vi "SVT Octave Analysis (N Ch).vi"(0 "scaled signals [EU]":waveform(dbl)[](array[waveform])=[{"t0"=timestamp(0 s since 1904-01-01), "dt"=1.0, "Y"=[]}], 1 "restart averaging (F)":bool, 2 "reset filter (F)":bool, 5 "frequency range":T7={"low band"=enum."16 Hz", "high band"=enum."16000 Hz"}, 9 "dB On (T)":bool=TRUE, 11 "error in (no error)":errorcluster, 12 "averaging type":T8(ring), 13 "exp avg settings":T1={" mode"=enum."Fast", "time constant [ms]"=125.0} {"time constant [ms]" format="%.2f"}, 14 "equal confidence level [dB]":dbl=125.0 format="%.2f") -> (3 "filter settled":bool, 4 "octave spectra":T6(array[cluster]) {"band power" format="%.2f"; "nominal frequencies [Hz]" format="%.2f"}, 6 "unit labels":string[](array[string]), 8 "total band powers":dbl[](array[numeric]) format="%.2f", 10 "octave info":T2[](array[typedef]) {"engineering units" items=["custom..."=0, "V"=1, "A"=21, "C"=30, "pC"=31, "s"=32, "-"=29, "Pa"=2, "N"=20, "g"=3, "m/s^2"=4, "m/s"=5, "m"=6, "mm/s"=12, "mm"=13, "micron/s"=14, "micron"=15, "in/s^2"=7, "in/s"=8, "in"=9, "mil/s"=10, "mil"=11, "rad/s^2"=16, "rad/s"=17, "rad"=18, "deg/s^2"=26, "deg/s"=27, "deg"=28, "RPM"=22, "cycle/s^2"=23, "Hz"=24, "cycle"=25, "strain"=19]; "dB reference" format="%.2e"; "weighting filter" items=["Linear", "A-weighting", "B-weighting", "C-weighting", "ITU-R 468-4", "Dolby", "CCITT", "C-message", "Wb", "Wc", "Wd", "We", "Wf", "Wh", "Wj", "Wk", "Wm", "AES17 20 kHz lowpass", "AES17 40 kHz lowpass", "AES17 20 kHz highpass", "AES17 40 kHz highpass"]}, 15 "error out":errorcluster)   [LabVIEW 2017, in "SoundVib_Octave.lvlib"]
doc: "LabVIEW no longer supports this VI. The SVT Octave Analysis VI is available for compatibility with previous versions of the LabVIEW Sound and Vibration Toolkit. This version of the SVT Octave Analysis VI performs an octave analysis on <B>scaled signal [EU]</B> in accordance with the IEC 1260 standard. This standard has been superseded by the new IEC 61260 standard. If you want to ensure compliance with the latter standard, use the SVT Octave Analysis VI, located on the Octave Analysis palette instead. You can use this polymorphic VI to perform octave analysis on a single channel or on N channels. The data type you wire to the <B>scaled signal [EU]</B> input determines the polymorphic instance to use."
uses:
  <vilib>/addons/Sound and Vibration/svt_Octave/SoundVib_Octave.lvlib
  <vilib>/addons/_NISVFA/_Shared subVIs/Controls/svc_Octave Info.ctl
  <vilib>/addons/_NISVFA/_Shared subVIs/Controls/svc_Octave Standard.ctl
  <vilib>/addons/_NISVFA/_Shared subVIs/Controls/svc_Weighting Filter Text Ring.ctl
  <vilib>/addons/_NISVFA/_Shared subVIs/Controls/svc_Engineering Units Text Ring.ctl
  <vilib>/addons/Sound and Vibration/svt_Octave_2014 standard/SoundVib_Octave_2014 standard.lvlib
panel:
  out "# samples to settle":u64
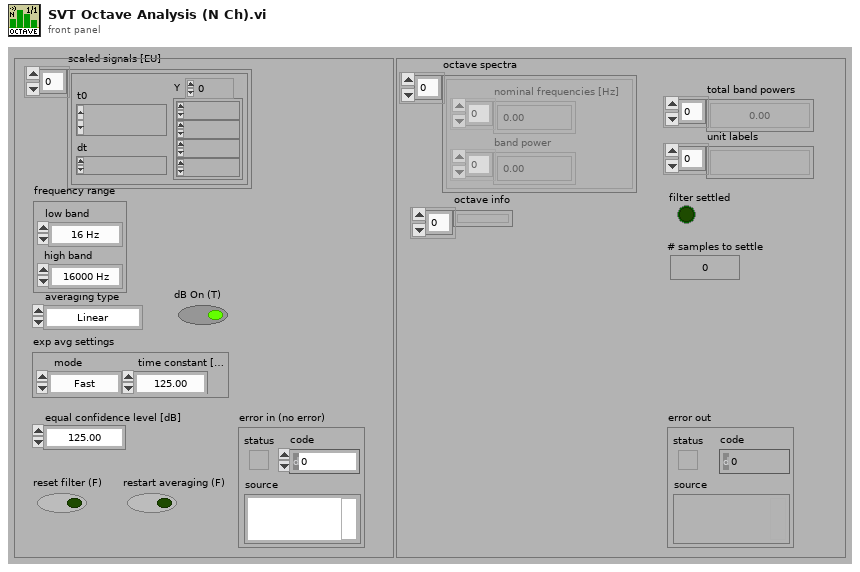
[diagram p1: front panel]
types:
  T1 = cluster{" mode":enum16{"Slow", "Fast", "Impulse", "Custom"}, "time constant [ms]":dbl}
  T2 = typedef "svc_Octave Info.ctl" = cluster{"standard":T3, "bandwidth":enum16{"1 octave", "1/3 octave", "1/6 octave", "1/12 octave", "1/24 octave"}, "low band":i32, "high band":i32, "weighting filter":T4, "dB reference":dbl, "dB On":bool, "unit label":string, "channel name":string, "description":string, "engineering units":T5, "custom label":string, "spectrum type":enum16{"power", "magnitude"}, "spectral density":bool, "filters settled":bool}
  T3 = typedef "svc_Octave Standard.ctl" = enum16{"ANSI S1.11", "IEC 61260"}
  T4 = typedef "svc_Weighting Filter Text Ring.ctl" = u16
  T5 = typedef "svc_Engineering Units Text Ring.ctl" = u16
  T6 = cluster{"nominal frequencies [Hz]":dbl[], "band power":dbl[]}[]
  T7 = cluster{"low band":enum16{"16 Hz", "31.5 Hz", "63 Hz", "125 Hz", "250 Hz", "500 Hz", "1000 Hz", "2000 Hz", "4000 Hz", "8000 Hz", "16000 Hz"}, "high band":enum16{"16 Hz", "31.5 Hz", "63 Hz", "125 Hz", "250 Hz", "500 Hz", "1000 Hz", "2000 Hz", "4000 Hz", "8000 Hz", "16000 Hz"}}
  T8 = enum16{"Linear", "Exponential", "Equal confidence", "Peak"}
  T9 = cluster{"standard":T3, "bandwidth":enum16{"1 octave", "1/3 octave", "1/6 octave", "1/12 octave", "1/24 octave"}}
  T10 = cluster{"dup nominal frequencies [Hz":dbl[], "band power [EU^2 rms]":dbl[]}[]
  T11 = cluster{"nominal frequencies [Hz]":dbl[], "band power [dB EU]":dbl[]}[]
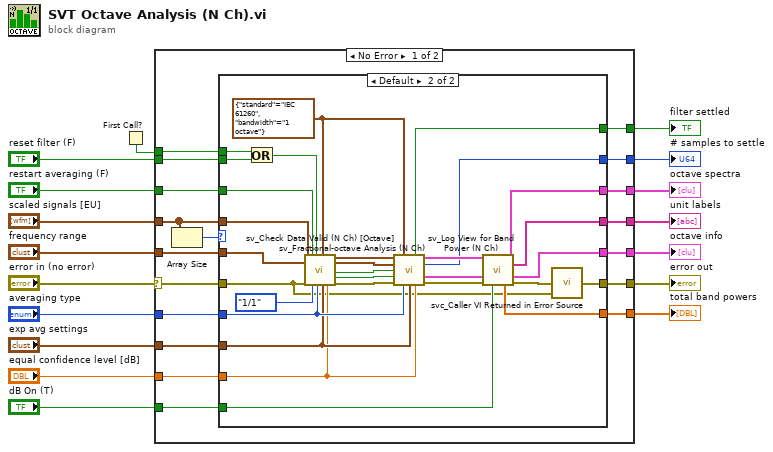
[diagram p0: block diagram]
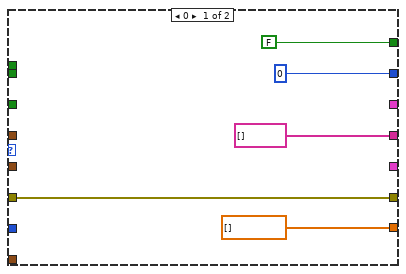
[diagram p2: hidden frame]
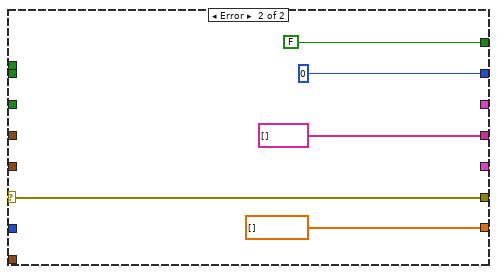
[diagram p3: hidden frame]
diagram:
  n1 = First Call?() -> (First Call?: T/F=w1:bool)
  n2 = case shown="No Error" "error in (no error)" {
    selector: "error in (no error)" -> [w25 w74]
    tunnel: "restart averaging (F)" -> [w35 _]
    tunnel: "frequency range" -> [w34 _]
    tunnel: [w23 FALSE ("settled?")] -> w15
    tunnel: "dB On (T)" -> [w33 _]
    tunnel: "averaging type" -> [w32 _]
    tunnel: "equal confidence level [dB]" -> [w24 _]
    tunnel: "exp avg settings" -> [w31 _]
    tunnel: [w30 dbl[] [] ("total band power(s) [dB EU]")] -> w10
    tunnel: "scaled signals [EU]" -> [w19 _]
    tunnel: [w26 w74] -> w8
    tunnel: [w29 _] -> w7
    tunnel: [w28 string[] [] ("unit labels")] -> w6
    tunnel: [w27 _] -> w5
    tunnel: [w22 u64 0 ("# samples to settle")] -> w3
    tunnel: "reset filter (F)" -> [w21 _]
    tunnel: w1 -> [w20 _]
    frame No Error {
      n3 = Array Size(array=w19) -> (size(s)=w18:i32)
      n4 = case shown="Default" w18 {
        tunnel: w35 -> [_ w69]
        tunnel: w34 -> [_ w68]
        tunnel: w33 -> [_ w63]
        tunnel: w32 -> [_ w61]
        tunnel: w31 -> [_ w60]
        tunnel: [dbl[] [] ("total band power(s) [dB EU]") w59] -> w30
        tunnel: w19 -> [_ w56]
        tunnel: [_ w54] -> w29
        tunnel: [string[] [] ("unit labels") w53] -> w28
        tunnel: [_ w52] -> w27
        tunnel: [w37 w50] -> w26
        tunnel: w25 -> [w37 w41]
        tunnel: w24 -> [_ w48]
        tunnel: [FALSE ("settled?") w45] -> w23
        tunnel: [u64 0 ("# samples to settle") w44] -> w22
        tunnel: w21 -> [_ w43]
        tunnel: w20 -> [_ w42]
        frame 0 {
        }
        frame Default {
          w58 = T9 {"standard"=enum."IEC 61260", "bandwidth"=enum."1 octave"} ("1/n Octave settings")
          n5 = Or(x=w42, y=w43) -> (x .or. y?=w46:bool)
          n6 = call <vilib>:"sv_Check Data Valid (N Ch) [Octave].vi"("Scaled signal(s)"=w56, "frequency range (1/1)"=w68, "error in (no error)"=w41, "restart averaging (F)"=w69, "bandwidth"=enum16{"1/1", "1/3", "1/n"}."1/1", "reset filter (F)"=w46, "averaging type"=w61, "1/n Octave settings"=w58, "exp avg settings"=w60, "equal confidence level [dB]"=w48) -> ("dup Scaled signal(s)"=w64:waveform(dbl)[], "band number"=w57:cluster{"low band":i32, "high band":i32}, "Restart averaging"=w66:bool, "Reset Filter"=w47:bool, "error out"=w67:errorcluster)  [unwired: 5 in]
          n7 = call <vilib>:"sv_Fractional-octave Analysis (N Ch).vi"("Scaled signal(s)"=w64, "1/n octave settings"=w58, "band number"=w57, "restart averaging (F)"=w66, "reset filter (F)"=w47, "error in (no error)"=w67, "averaging type"=w61, "exp avg settings"=w60, "equal confidence level [dB]"=w48) -> ("settled?"=w45:bool, "Octave measurements"=w62:T10, "# samples to settle"=w44:u64, "octave info"=w51:T2[], "error out"=w65:errorcluster)  [unwired: 2 in]
          n8 = call <vilib>:"sv_Log View for Band Power (N Ch).vi"("Octave measurements"=w62, "octave info"=w51, "error in (no error)"=w65, "dB On (T)"=w63) -> ("octave spectra"=w52:T11, "unit labels"=w53:string[], "octave info"=w54:T2[], "total band power(s) [dB EU]"=w59:dbl[], "error out"=w55:errorcluster)  [unwired: 7 in]
          n9 = call <vilib>:"svc_Caller VI Returned in Error Source.vi"("warning input to caller"=w41, "error in (no error)"=w55) -> ("error out"=w50:errorcluster)  [unwired: 3 in]
        }
      }
    }
    frame Error {
    }
  }
  "filter settled" <- w15
  "unit labels" <- w6
  "total band powers" <- w10
  "error out" <- w8
  "octave spectra" <- w5
  "octave info" <- w7
  "# samples to settle" <- w3
